vi "Resize window to image size.vi"(9 "Image":T1, 11 "Window VI's Ref":refnum<vi>) -> ()   [LabVIEW 2020]
uses:
  <vilib>/vision/Image Controls.llb/IMAQ Image.ctl
panel:
  in  "Y Boundaries size":i16=120
  in  "X Boundaries size":i16=100
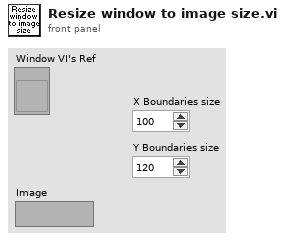
[diagram p1: front panel]
types:
  T1 = typedef "IMAQ Image.ctl" = refnum<image>
  T2 = typedef "LVRectTypeDef.ctl" = cluster{"Left":i16, "Top":i16, "Right":i16, "Bottom":i16}
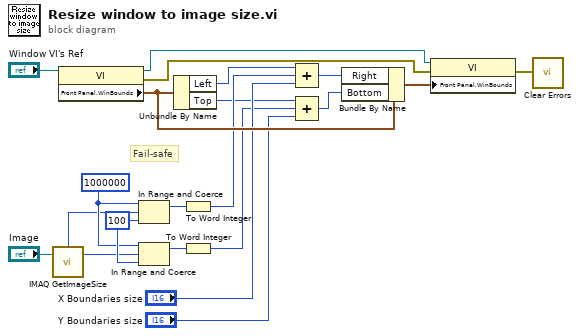
[diagram p0: block diagram]
diagram:
  w8 = 100 ("lower limit")
  w7 = 1000000 ("upper limit")
  # "Fail-safe"
  n1 = call "IMAQ GetImageSize"("Image"="Image") -> ("Y Resolution"=w6:i32, "X Resolution"=w5:i32)  [unwired: 3 in, 1 out]
  n2 = property class="VI"(reference="Window VI's Ref") -> (reference out=w20:refnum<vi>, error out=w2:errorcluster, "Front Panel.WinBounds"=w21:T2)  [unwired: 1 in]
  n3 = In Range and Coerce(upper limit=w7, x=w5, lower limit=w8) -> (coerced(x)=w12:i32)  [unwired: 1 out]
  n4 = In Range and Coerce(upper limit=w7, x=w6, lower limit=w8) -> (coerced(x)=w13:i32)  [unwired: 1 out]
  n5 = Unbundle By Name(w21) -> ("Left"=w10:i16, "Top"=w11:i16)
  n6 = To Word Integer(number=w12) -> (16bit integer=w16:i16)
  n7 = To Word Integer(number=w13) -> (16bit integer=w17:i16)
  n8 = Compound Arithmetic op=ADD(w10, w16, "X Boundaries size") -> (w14:i16)
  n9 = Compound Arithmetic op=ADD(w11, w17, "Y Boundaries size") -> (w15:i16)
  n10 = Bundle By Name(cluster=w21, "Right"=w14, "Bottom"=w15) -> (w19:T2)
  n11 = property class="VI"(reference=w20, error in=w2, "Front Panel.WinBounds"=w19) -> (error out=w3:errorcluster)  [unwired: 1 out]
  n12 = call <vilib>:"Clear Errors.vi"("error in (no error)"=w3) -> ()  [unwired: 5 in, 2 out]
